vi "Execute.vi"(5 "Init user event out":refnum<user-event>, 7 "user event in":refnum<user-event>, 8 "Advanced Waveform In":refnum<class "Advanced Waveform.lvclass">, 9 "FFT Signal Message in":refnum<class "FFT Signal Message.lvclass">, 10 "Command Queue":refnum<queue>, 11 "error in (no error)":errorcluster) -> (0 "Advanced Waveform Out":refnum<class "Advanced Waveform.lvclass">, 1 "FFT Signal Message out":refnum<class "FFT Signal Message.lvclass">, 2 "Stop":bool, 3 "error out":errorcluster)   [LabVIEW 2011, in "FFT Signal Message.lvclass"]
uses:
  FFT Signal Message.lvclass
  Advanced Waveform Class/Advanced Waveform.lvclass
  Message.lvclass
  Display Message/Display Message.lvclass
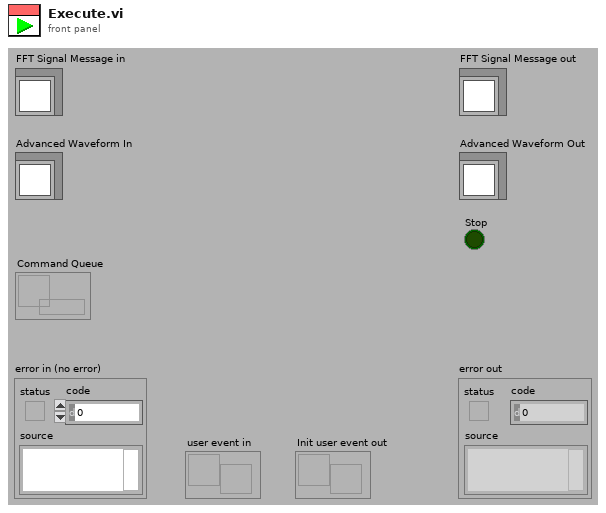
[diagram p1: front panel]
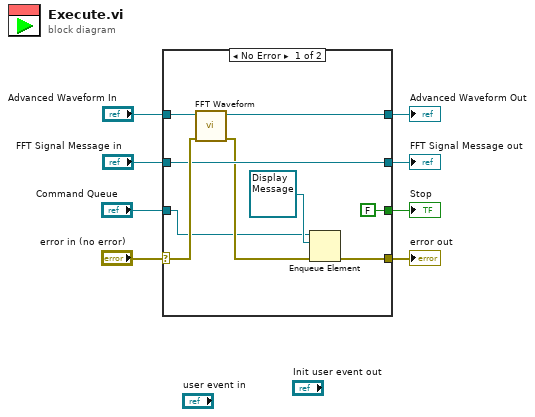
[diagram p0: block diagram]
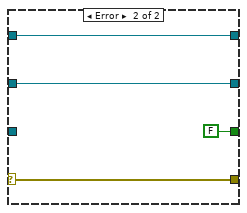
[diagram p2: hidden frame]
diagram:
  n1 = case shown="No Error" "error in (no error)" {
    selector: "error in (no error)" -> [w15 w21]
    tunnel: "Command Queue" -> [w9 _]
    tunnel: "FFT Signal Message in" -> [w13 w18]
    tunnel: "Advanced Waveform In" -> [w16 w19]
    tunnel: [w12 w21] -> w4
    tunnel: [FALSE FALSE] -> w3
    tunnel: [w14 w19] -> w2
    tunnel: [w13 w18] -> w1
    frame No Error {
      n2 = call-dynamic "FFT Waveform.vi"("error in (no error)"=w15, "Waveform in"=w16) -> ("error out"=w11:errorcluster, "Waveform out"=w14:refnum<class "Advanced Waveform.lvclass">)  [unwired: 8 in]
      n3 = Enqueue Element(queue=w9, element=refnum<class "Display Message.lvclass"> refnum ("Display Message.lvclass"), error in (no error)=w11) -> (error out=w12:errorcluster)  [unwired: 1 in, 2 out]
    }
    frame Error {
    }
  }
  "error out" <- w4
  "FFT Signal Message out" <- w1
  "Stop" <- w3
  "Advanced Waveform Out" <- w2
